vi "Other Connected Terminal.vi"(8 "error in (no error)":errorcluster, 10 "Terminal":refnum<vi>) -> (0 "error out":errorcluster, 2 "Other":refnum<vi>)   [LabVIEW 2020, in "LV-Protoc.lvlib"]
uses:
  LV-Protoc.lvlib
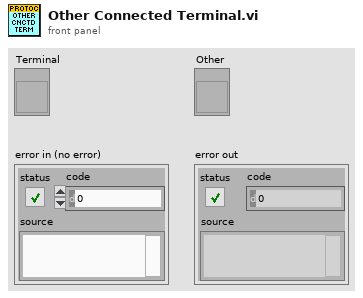
[diagram p1: front panel]
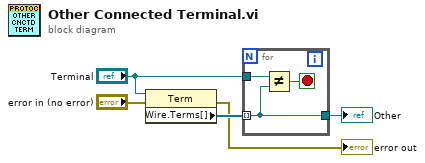
[diagram p0: block diagram]
diagram:
  n1 = property class="Term"(reference="Terminal", error in="error in (no error)") -> (error out=→"error out":errorcluster, "Wire.Terms[]"=w4:refnum<vi>[])  [unwired: 1 out]
  n2 = for {
    tunnel: w4 -> [w7] mode=indexing
    tunnel: "Terminal" -> [w8]
    tunnel: [w7] -> w1
    stop <- w6 stop-if-true
    n3 = Not Equal?(x=w8, y=w7) -> (x != y?=w6:bool)
  }
  "Other" <- w1
